vi "Fehler nach Tabelle.vi"(10 "Fehler":T1[](array[typedef]) {"level" items=["Geringfügiger Fehler", "Schwerer Fehler", "Nicht behebbarer Fehler"]}) -> (2 "Tabelle Fehler":string[](array[string]))   [LabVIEW 2020, in "cRIO Ueberwachung.lvlib"]
uses:
  cRIO Ueberwachung.lvlib
  Fehler.ctl
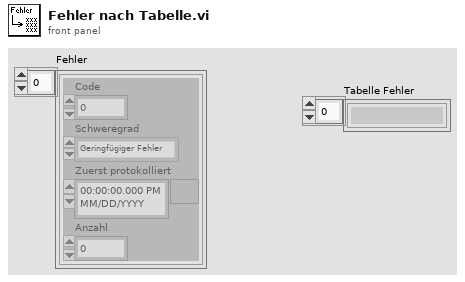
[diagram p1: front panel]
types:
  T1 = typedef "cRIO Ueberwachung.lvlib/Fehler.ctl" = cluster{"code":i32, "level":i32, "first reported time":timestamp, "number reported":u32}
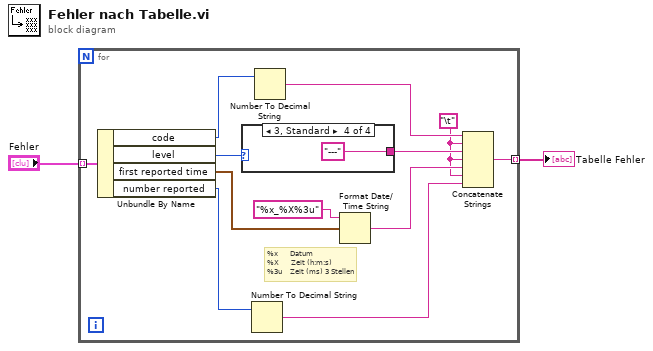
[diagram p0: block diagram]
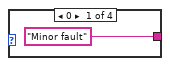
[diagram p2: hidden frame]
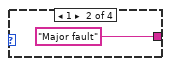
[diagram p3: hidden frame]
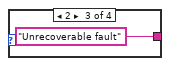
[diagram p4: hidden frame]
diagram:
  n1 = for {
    tunnel: "Fehler" -> [w9] mode=indexing
    tunnel: [w3] -> w1 mode=indexing
    w5 = "\t"
    # "%x      Datum\n%X      Zeit (h:m:s)\n%3u    Zeit (ms) 3 Stellen"
    n2 = Unbundle By Name(w9) -> ("code"=w14:i32, "level"=w13:i32, "first reported time"=w11:timestamp, "number reported"=w10:u32)
    n3 = case shown="3, Standard" w13 {
      tunnel: ["Minor fault" "Major fault" "Unrecoverable fault" "---"] -> w7
      frame 0 {
      }
      frame 1 {
      }
      frame 2 {
      }
      frame 3, Default {
      }
    }
    n4 = Number To Decimal String(number=w10) -> (decimal integer string=w4:string)  [unwired: 1 out]
    n5 = Number To Decimal String(number=w14) -> (decimal integer string=w8:string)  [unwired: 1 out]
    n6 = Format Date/Time String(time format string (%c)="%x_%X%3u" ("Zeitformatierungs-String (%c)"), seconds (now)=w11) -> (date/time string=w6:string)  [unwired: 1 in]
    n7 = Concatenate Strings(w8, w5, w7, w5, w6, w5, w4) -> (w3:string)
  }
  "Tabelle Fehler" <- w1
